vi "writeU32.vi"(8 "error in (no error)":errorcluster, 10 "Input":u32, 11 "ModbusBuffer in":refnum<class "ModbusBuffer.lvclass">) -> (0 "error out":errorcluster, 3 "ModbusBuffer out":refnum<class "ModbusBuffer.lvclass">)   [LabVIEW 2016, in "RTModbus.lvlib" / "ModbusBuffer.lvclass"]
uses:
  ModbusBuffer.lvclass
  ModbusBuffer.lvclass/ModbusBuffer.ctl
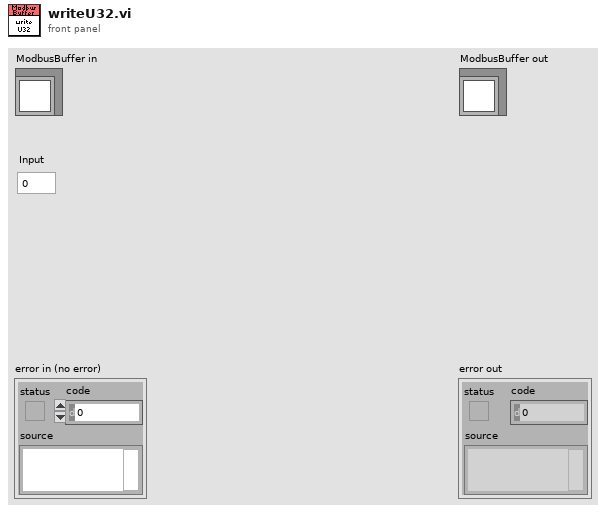
[diagram p1: front panel]
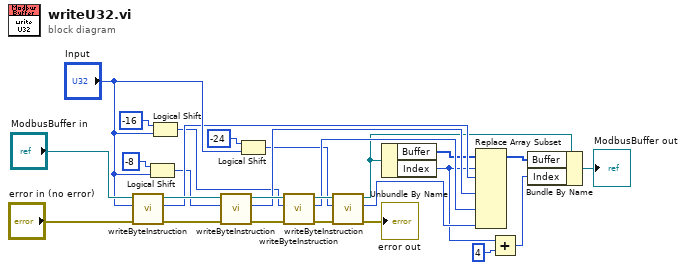
[diagram p0: block diagram]
diagram:
  n1 = call "writeByteInstruction.vi"("error in (no error)"="error in (no error)", "Input"="Input", "ModbusBuffer in"="ModbusBuffer in") -> ("error out"=w8:errorcluster, "Output"=w16:u16, "ModbusBuffer out"=w20:refnum<class "ModbusBuffer.lvclass">)  [unwired: 6 in]
  n2 = Logical Shift(y=i16 -8, x="Input") -> (x << y=w14:u32)
  n3 = Logical Shift(y=i16 -16, x="Input") -> (x << y=w13:u32)
  n4 = call "writeByteInstruction.vi"("error in (no error)"=w8, "Input"=w14, "ModbusBuffer in"=w20) -> ("error out"=w7:errorcluster, "Output"=w15:u16, "ModbusBuffer out"=w19:refnum<class "ModbusBuffer.lvclass">)  [unwired: 6 in]
  n5 = Logical Shift(y=i16 -24, x="Input") -> (x << y=w10:u32)
  n6 = call "writeByteInstruction.vi"("error in (no error)"=w7, "Input"=w13, "ModbusBuffer in"=w19) -> ("error out"=w6:errorcluster, "Output"=w12:u16, "ModbusBuffer out"=w18:refnum<class "ModbusBuffer.lvclass">)  [unwired: 6 in]
  n7 = call "writeByteInstruction.vi"("error in (no error)"=w6, "Input"=w10, "ModbusBuffer in"=w18) -> ("error out"=→"error out":errorcluster, "Output"=w11:u16, "ModbusBuffer out"=w5:refnum<class "ModbusBuffer.lvclass">)  [unwired: 6 in]
  n8 = Unbundle By Name(w5) -> ("Buffer"=w3:u16[], "Index"=w2:i32)
  n9 = Replace Array Subset(array=w3, new element #1=w16, index #1=w2, new element #2=w15, new element #3=w12, new element #4=w11) -> (w22:u16[])  [unwired: 3 in]
  n10 = Add(x=w2, y=4) -> (x+y=w26:i32)
  n11 = Bundle By Name(cluster=w5, "Buffer"=w22, "Index"=w26) -> (→"ModbusBuffer out":refnum<class "ModbusBuffer.lvclass">)
